vi "I2C Write Read.vi"(7 "Bytes to Read (1)":i32=1, 8 "error in (no error)":errorcluster, 9 "I2C Address (0x70)":i32=112 format="%x", 10 "Data":u8[](array[numeric])=[0] format="%x", 11 "I2C Task In":T1) -> (0 "error out":errorcluster, 2 "Data Out":u8[](array[numeric]) format="%x", 3 "I2C Task Out":T1)   [LabVIEW 2017, in "I2C.lvlib"]
doc: "Writes the specified number of bytes from <b>Data</b> to the specified address and returns <b>Bytes to Read</b> number of bytes, most significant bit first. The I2C address is actually a 7-bit I2C address with an expansion of one 0 at the highest bit."
uses:
  <vilib>/robotics/Protocols/I2C/DAQmx/I2C.lvlib
  <vilib>/robotics/Protocols/I2C/DAQmx/Private/I2C Tasks.ctl
panel:
  # "The I2C address is actually a 7-bit I2C address with an expansion of one 0 at the highest bit."
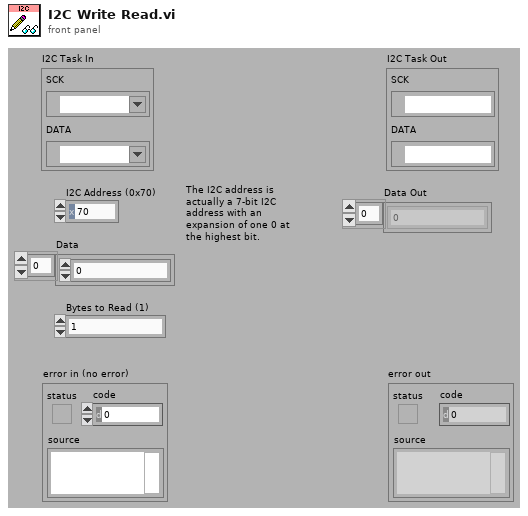
[diagram p1: front panel]
types:
  T1 = typedef "I2C.lvlib/I2C Tasks.ctl" = cluster{"SCK":refnum<k21>, "DATA":refnum<k21>}
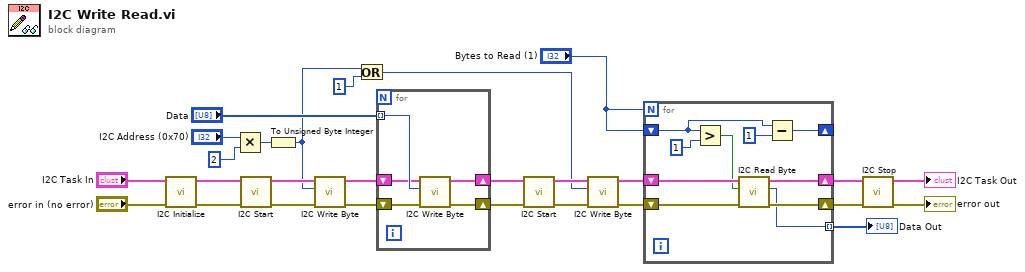
[diagram p0: block diagram]
diagram:
  n1 = call <vilib>:"I2C Initialize.vi"("error in (no error)"="error in (no error)", "I2C Task In"="I2C Task In") -> ("error out"=w24:errorcluster, "I2C Task Out"=w25:T1)  [unwired: 8 in]
  n2 = Multiply(x="I2C Address (0x70)", y=2) -> (x*y=w21:i32)
  n3 = call <vilib>:"I2C Start.vi"("error in (no error)"=w24, "I2C Task In"=w25) -> ("error out"=w19:errorcluster, "I2C Task Out"=w20:T1)  [unwired: 8 in]
  n4 = To Unsigned Byte Integer(number=w21) -> (unsigned 8bit integer=w13:u8)
  n5 = call <vilib>:"I2C Write Byte.vi"("error in (no error)"=w19, "Data Byte (0x0)"=w13, "I2C Task In"=w20) -> ("error out"=w17:errorcluster, "I2C Task Out"=w18:T1)  [unwired: 6 in, 1 out]
  n6 = Or(x=w13, y=u8 1) -> (x .or. y?=w9:u8)
  n7 = for {
    shift-right: [w29] -> w15
    shift-left: w18 -> [w31]
    shift-right: [w28] -> w14
    shift-left: w17 -> [w30]
    tunnel: "Data" -> [w32] mode=indexing
    n8 = call <vilib>:"I2C Write Byte.vi"("error in (no error)"=w30, "Data Byte (0x0)"=w32, "I2C Task In"=w31) -> ("error out"=w28:errorcluster, "I2C Task Out"=w29:T1)  [unwired: 6 in, 1 out]
  }
  n9 = call <vilib>:"I2C Start.vi"("error in (no error)"=w14, "I2C Task In"=w15) -> ("error out"=w10:errorcluster, "I2C Task Out"=w11:T1)  [unwired: 8 in]
  n10 = call <vilib>:"I2C Write Byte.vi"("error in (no error)"=w10, "Data Byte (0x0)"=w9, "I2C Task In"=w11) -> ("error out"=w7:errorcluster, "I2C Task Out"=w8:T1)  [unwired: 6 in, 1 out]
  n11 = for {
    N: "Bytes to Read (1)" -> [_]
    shift-right: [w36] -> _
    shift-left: "Bytes to Read (1)" -> [w38]
    shift-right: [w35] -> w4
    shift-left: w8 -> [w42]
    shift-right: [w34] -> w3
    shift-left: w7 -> [w41]
    tunnel: [w33] -> w5 mode=indexing
    n12 = Greater?(x=w38, y=1) -> (0:w39:bool)
    n13 = call <vilib>:"I2C Read Byte.vi"("error in (no error)"=w41, "Ack? (F:False)"=w39, "I2C Task In"=w42) -> ("error out"=w34:errorcluster, "Data Byte"=w33:u8, "I2C Task Out"=w35:T1)  [unwired: 6 in]
    n14 = Subtract(x=w38, y=1) -> (x-y=w36:i32)
  }
  "Data Out" <- w5
  n15 = call <vilib>:"I2C Stop.vi"("error in (no error)"=w3, "I2C Task In"=w4) -> ("error out"=→"error out":errorcluster, "I2C Task Out"=→"I2C Task Out":T1)  [unwired: 8 in]
